vi "Create file.vi"(0 "reference in":refnum<class "TDMS_DataHandler.lvclass">, 2 "TDMS filename":string, 5 "error in (no error)":errorcluster) -> (14 "reference out":refnum<class "TDMS_DataHandler.lvclass">, 15 "tdms file out":refnum<k34>, 19 "error out":errorcluster)   [LabVIEW 2019, in "TDMS_DataHandler.lvclass"]
uses:
  TDMS_DataHandler.lvclass
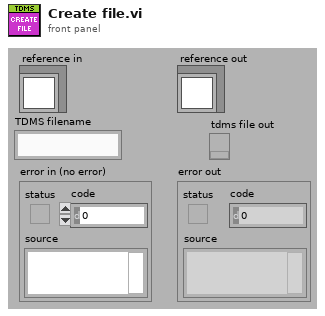
[diagram p1: front panel]
types:
  T1 = enum16{"open", "open or create", "create or replace", "create", "open (read-only)"}
  T2 = typedef "TDMS_DataHandler.lvclass/ObjectAttributesRef.ctl" = refnum<data-value>
  T3 = typedef "TDMS_DataHandler.lvclass/ObjectAttributes.ctl" = cluster{"Directory":path, "FilePath":path, "FileRef":refnum<k34>, "ExperimentName":string, "GroupName":string, "ChannelNames":string[], "Datum":waveform(dbl)[], "Group_Metadata":cluster{"property names":string[], "property values":variant[]}, "Channel_Metadata":cluster{"property names":string[], "property values":variant[]}}
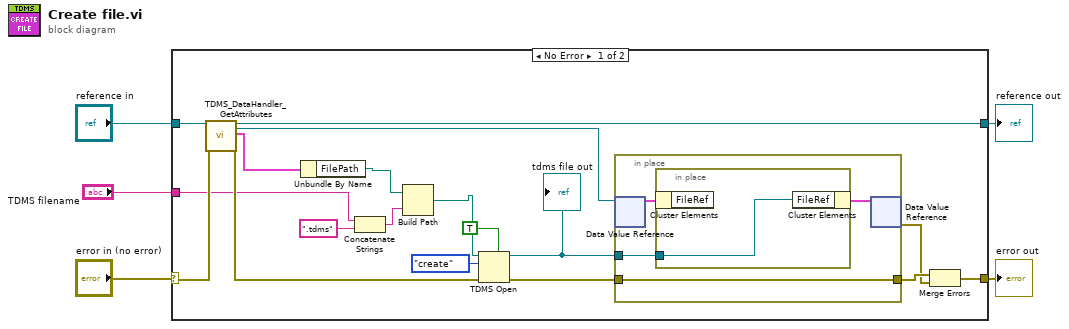
[diagram p0: block diagram]
diagram:
  n1 = case shown="No Error" "error in (no error)" {
    selector: "error in (no error)" -> [w21 w30]
    tunnel: [w23 w30] -> w4
    tunnel: [w16 w29] -> w2
    tunnel: "reference in" -> [w22 w29]
    tunnel: "TDMS filename" -> [w6 _]
    frame No Error {
      n2 = call "TDMS_DataHandler_GetAttributes.vi"("reference in"=w22, "error in (no error)"=w21) -> ("reference out"=w16:refnum<class "TDMS_DataHandler.lvclass">, "attributes ref"=w18:T2, "attributes"=w17:T3, "error out"=w15:errorcluster)  [unwired: 14 in]
      n3 = Unbundle By Name(w17) -> ("FilePath"=w10:path)
      n4 = Concatenate Strings(w6, ".tdms" ("string")) -> (w8:string)
      n5 = Build Path(base path=w10, name or relative path=w8) -> (appended path=w9:path)
      n6 = TDMS Open(5:TRUE ("create index file? (T)"), 8:w15, 10:T1."create" ("operation (0:open)"), 11:w9) -> (0:w14:errorcluster, 3:w13:refnum<k34>)  [unwired: 3 in]
      "tdms file out" <- w13
      n7 = in-place {
        in-place-border: w14 -> [w25]
        in-place-border: [w25] -> w20
        in-place-border: w13 -> [w24]
        n8 = in-place-dvr #1(w18) -> (w26:T3)  [unwired: 1 out]
        n9 = in-place {
          in-place-border: w24 -> [w28]
          n10 = in-place-cluster #2(w26) -> ()  [unwired: 1 out]
          n11 = in-place-cluster #2("FileRef"=w28) -> (w27:T3)
        }
        n12 = in-place-dvr #1(w27) -> (w19:errorcluster)  [unwired: 1 out]
      }
      n13 = Merge Errors(w20, w19) -> (w23:errorcluster)
    }
    frame Error {
    }
  }
  "error out" <- w4
  "reference out" <- w2
